vi "AutoSteering.vi"(8 "Captured Num Long":i32, 9 "Captured Num Lat":i32) -> (1 "Steer":dbl)   [LabVIEW 2011]
panel:
  out "Theoretical Y":dbl format="%#_20f"
  out "Move counts":dbl format="%#_15g"
  out "Error":dbl
  out "Delta Y":dbl format="%#_20f"
  out "Delta X":dbl
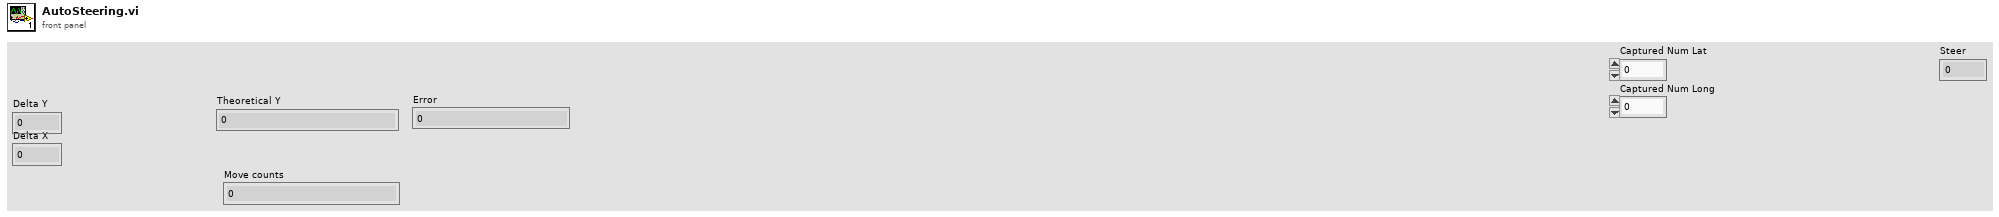
[diagram p1: front panel]
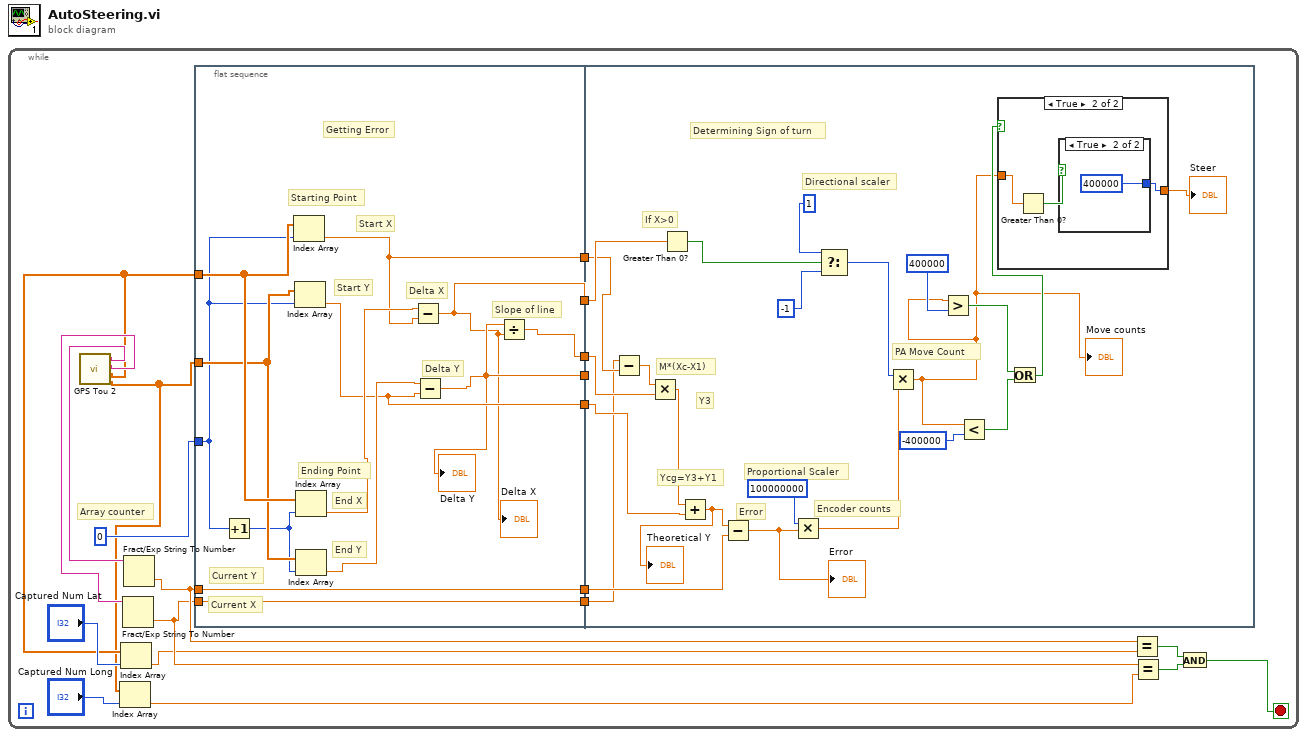
[diagram p0: block diagram]
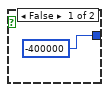
[diagram p3: hidden frame]
diagram:
  n1 = while {
    stop <- w5 stop-if-true
    # "Array counter"
    n2 = call "GPS Tou 2.vi"() -> ("Captured Longitude"=w1:dbl[], "Captured Latitude"=w2:dbl[], "Current Longitude (xx deg, xxxxxx min)"=w3:string, "Current Latitude (xx deg, xxxxxx min)"=w4:string)  [unwired: 7 in, 1 out]
    n3 = Index Array(array=w1, index="Captured Num Long") -> (element=w9:dbl)
    n4 = Index Array(array=w2, index="Captured Num Lat") -> (element=w8:dbl)
    n5 = Fract/Exp String To Number(string=w3) -> (number=w10:dbl)  [unwired: 3 in, 1 out]
    n6 = Fract/Exp String To Number(string=w4) -> (number=w11:dbl)  [unwired: 3 in, 1 out]
    n7 = flat-sequence {
      tunnel: w2 -> [w34]
      tunnel: w1 -> [w33]
      tunnel: 0 -> [w32]
      tunnel: [w25] -> w21
      tunnel: [w26] -> w20
      tunnel: [w27] -> w19
      tunnel: [w28] -> w18
      tunnel: [w24] -> w17
      tunnel: [w23] -> w16
      tunnel: w11 -> [w23]
      tunnel: [w22] -> w15
      tunnel: w10 -> [w22]
      tunnel: w21 -> [w45]
      tunnel: w20 -> [_]
      tunnel: w19 -> [w44]
      tunnel: w18 -> [w42]
      tunnel: w17 -> [w40]
      tunnel: w16 -> [w37]
      tunnel: w15 -> [w36]
      frame #0 {
        # "End Y"
        # "End X"
        # "Start Y"
        # "Start X"
        # "Current X"
        # "Current Y"
        # "Getting Error"
        # "Slope of line"
        # "Delta Y"
        # "Delta X"
        # "Ending Point"
        # "Starting Point"
        n8 = Increment(x=w32) -> (x+1=w31:i32)
        n9 = Index Array(array=w34, index=w32) -> (element=w24:dbl)
        n10 = Index Array(array=w33, index=w32) -> (element=w27:dbl)
        n11 = Index Array(array=w34, index=w31) -> (element=w29:dbl)
        n12 = Index Array(array=w33, index=w31) -> (element=w30:dbl)
        n13 = Subtract(x=w29, y=w24) -> (x-y=w25:dbl)
        "Delta X" <- w25
        n14 = Subtract(x=w30, y=w27) -> (x-y=w26:dbl)
        "Delta Y" <- w26
        n15 = Divide(x=w26, y=w25) -> (x/y=w28:dbl)
      }
      frame #1 {
        # "Y3"
        # "Ycg=Y3+Y1"
        # "M*(Xc-X1)"
        # "PA Move Count"
        # "Directional scaler"
        # "Encoder counts"
        # "Proportional Scaler"
        # "Error"
        # "If X>0"
        # "Determining Sign of turn"
        n16 = Subtract(x=w36, y=w40) -> (x-y=w41:dbl)
        n17 = Multiply(x=w41, y=w42) -> (x*y=w43:dbl)
        n18 = Greater Than 0?(x=w45) -> (x > 0?=w47:bool)
        n19 = Add(x=w43, y=w44) -> (x+y=w39:dbl)
        "Theoretical Y" <- w39
        n20 = Subtract(x=w39, y=w37) -> (x-y=w38:dbl)
        "Error" <- w38
        n21 = Multiply(x=100000000, y=w38) -> (x*y=w53:dbl)
        n22 = Select(t=1, s=w47, f=-1) -> (s? t:f=w54:i32)
        n23 = Multiply(x=w54, y=w53) -> (x*y=w46:dbl)
        "Move counts" <- w46
        n24 = Greater?(x=w46, y=400000) -> (0:w50:bool)
        n25 = Less?(x=w46, y=-400000) -> (x < y?=w49:bool)
        n26 = Or(x=w50, y=w49) -> (x .or. y?=w48:bool)
        n27 = case shown="True" w48 {
          tunnel: w46 -> [w58 w61]
          tunnel: [w58 w59] -> w35
          frame False {
          }
          frame True {
            n28 = Greater Than 0?(x=w61) -> (x > 0?=w60:bool)
            n29 = case shown="True" w60 {
              tunnel: [-400000 400000] -> w59
              frame False {
              }
              frame True {
              }
            }
          }
        }
        "Steer" <- w35
      }
    }
    n30 = Equal?(x=w11, y=w8) -> (x = y?=w13:bool)
    n31 = Equal?(x=w10, y=w9) -> (x = y?=w12:bool)
    n32 = And(x=w13, y=w12) -> (x .and. y?=w5:bool)
  }
